vi "GetNI_SaveToFile.vi"(0 "Digitizer Settings":T5={"Digitizer delay (us) "=0.0, "rf points per line"=2048, "lines per plane"=128, "Samp Rate (Hz)"=100000000.0, "Additional dig delay (us)"=0.0, "Voltage Scale"=0.4, "Pre-Looks"=0, "Offset delay (us)"=0.0, "bits A/D"=8, "Avg Num"=1, "DigTimeOut"=5.0, "Rel Dig Delay"=0.0, "Dig Ch"=0, "LeCroyCluster"={"LeCroy Channels"=[TRUE, FALSE, FALSE, FALSE], "LC read pt offset"=0.0, "Sweep Avg"=FALSE}, "Main Digitizer"=enum."NI Digitizer", "Dig Config"=enum."Single channel", "Digitizer ID Cluster"={"Acqiris/Alazar/SP ID"=[], "NI Instr Handles"=[], "LeCroy VISA"="", "GaGe Handle"={"Handle"=0, "Sample size"=0, "Resolution"=0, "Offset"=0, "Channels"=0, "Boards"=0}, "ATS Ref"="ATS9350", "Acqiris Address"=["PCI::INSTR0"], "ADQRef"=refnum, "adq_cu_ptr"=refnum}, "Trigger Settings"={"Trig Source"=1, "Trig Coupling"=0, "Trig Slope"=0, "Level (mV)"=1500.0}, "Bulk Acq"=FALSE, "Bulk Start Indexes"=[], "Data Ref RF"=refnum, "NI ID/Channel"=[], "Total Dig CH"=1, "Xtra Ann Trig delay (us)"=10.0, "Fix Z Delay?"=FALSE, "One Way Transmission?"=FALSE, "Data Ref Log"=refnum} {"Trigger Settings"."Trig Slope" items=["Positive", "Negative"]; "Trigger Settings"."Level (mV)" format="%.2f"; "Trigger Settings"."Trig Coupling" items=["DC 1 MOhm", "AC 1 MOhm", "DC 50 Ohm", "AC 50 Ohm"]; "Trigger Settings"."Trig Source" items=["Chan 1", "External"]; "Rel Dig Delay" format="%.2f"; "DigTimeOut" format="%.2f"; "Avg Num" min=1; "Offset delay (us)" format="%.2f"; "Additional dig delay (us)" format="%.2f"; "Digitizer delay (us)" format="%.2f"}, 3 "NI Card":refnum<k15>, 6 "Motion Settings":T1={"No Motion?"=FALSE, "Motion System"=enum."NI 735x", "Motion Bd ID"=1, "Motion Profile"="SMAC1", "# Axis"=1, "Reverse Z axis?"=TRUE, "SMAC Axis"=0, "scan pair"=enum."y-(x) scan", "RT fps"=6.0, "Steps per mm"=[1000, 1000, 1000, 1000], "Motor Parameters"={"velocity ct/s"=[10000.0, 10000.0, 10000.0, 50000.0], "accel ct/s^2"=[50000.0, 50000.0, 50000.0, 200000.0]}, "One Way Scan"=FALSE, "Reverse One Way Scan"=FALSE, "Global Position (mm)"=[], "Plane"=0, "Distance between\nscan lines (um)"=0.0, "Distance between\nscan planes (um)"=0.0, "number of scan planes"=1, "Total steps in line"=0, "Xtra plane\ndistance  (um)"=100, "Xtra planes "=1, "Add Axis"=FALSE, "overshoot cts"=200, "BKPT Shift"=0, "Scan Start Time (ms)"=0, "ESP VISA"="GPIB::1::INSTR", "3rd Axis"=1, "GL Ref Out"=refnum, "Galil Address"=""} {"3rd Axis" items=["x", "y", "z", "w"]; "Xtra planes" min=1; "Xtra plane\ndistance  (um)" min=0; "Distance between\nscan planes (um)" format="%.2f"; "Distance between\nscan lines (um)" format="%.2f"; "SMAC Axis" items=["None"=0, "Axis 1"=1, "Axis 2"=2, "Axis 3"=3, "Axis 4"=4, "Axis 5"=5, "Axis 6"=6, "Axis 7"=7, "Axis 8"=8, "Vector Space 1"=17, "Vector Space 2"=18, "Vector Space 3"=19, "Vector Space 4"=20]; "Motion Bd ID" min=1 max=32 step=1}, 7 "errorin":errorcluster, 8 "File Array":string[](array[string]), 9 "Pulser Channel":i32, 10 "lines per plane":i32, 12 "Start Record":i32, 15 "Reverse?":bool) -> (17 "Raw VGain (scale)":dbl, 18 "Gain Array":T9(array[cluster]), 21 "VGain (dB)":dbl, 27 "error out":errorcluster)   [LabVIEW 2022 SP3]
uses:
  -DigitizerRoutines/DigitizerSettings.ctl
  -DigitizerRoutines/Digitizer.ctl
  -DigitizerRoutines/DigConfig.ctl
  -DigitizerRoutines/DigitizerID.ctl
  C:/Windows/System32/ADQAPI_dotNet_helper.dll
  Motion Controllers/NI_controller/-NI_MotionRoutines/MotionParameters.ctl
  Motion Controllers/NI_controller/-NI_MotionRoutines/MotionSys.ctl
  Motion Controllers/-MotionRoutines/ScanAxis.ctl
  Motion Controllers/-MotionRoutines/3rdAxis.ctl
  <instrlib>/niScope/Acquire/Fetch/niScope Multi Fetch Binary 8.vi
  -ScanSystem/DataHandling/ReverseDataI8.vi
panel:
  # "1-D and 2-D B scan settings"
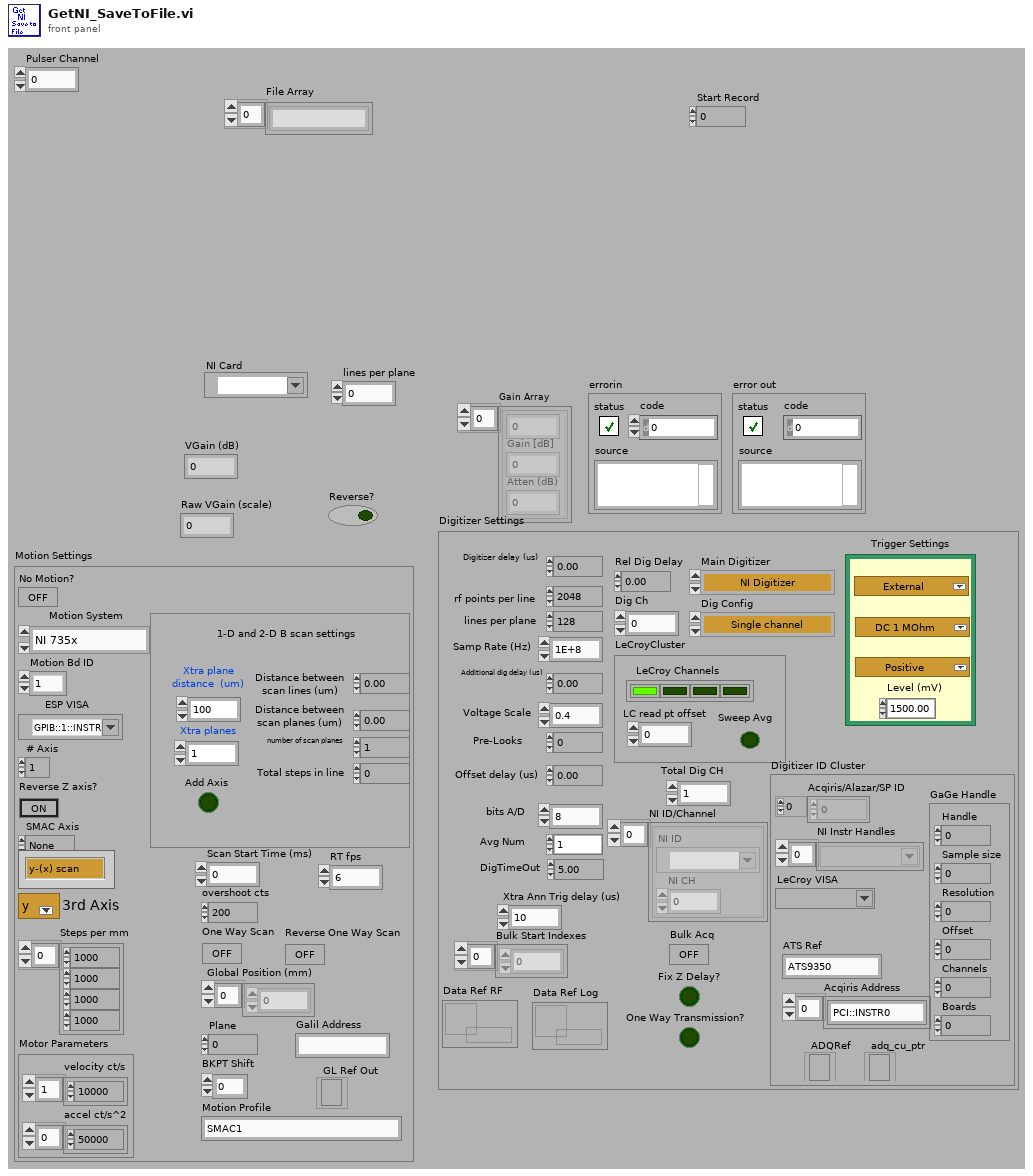
[diagram p1: front panel]
types:
  T1 = typedef "MotionParameters.ctl" = cluster{"No Motion?":bool, "Motion System":T2, "Motion Bd ID":u8, "Motion Profile":string, "# Axis":i8, "Reverse Z axis?":bool, "SMAC Axis":u16, "scan pair":T3, "RT fps":sgl, "Steps per mm":i32[], "Motor Parameters":cluster{"velocity ct/s":dbl[], "accel ct/s^2":dbl[]}, "One Way Scan":bool, "Reverse One Way Scan":bool, "Global Position (mm)":dbl[], "Plane":i32, "Distance between\nscan lines (um)":sgl, "Distance between\nscan planes (um)":sgl, "number of scan planes":i32, "Total steps in line":i32, "Xtra plane\ndistance  (um)":i32, "Xtra planes ":i32, "Add Axis":bool, "overshoot cts":i32, "BKPT Shift":i32, "Scan Start Time (ms)":u32, "ESP VISA":refnum<visa-resource-name>, "3rd Axis":T4, "GL Ref Out":refnum<k7>, "Galil Address":string}
  T2 = typedef "MotionSys.ctl" = enum16{"MM3000", "NI 735x", "Newport ESP", "No Motion Card", "Galil"}
  T3 = typedef "ScanAxis.ctl" = enum16{"y-(x) scan", "x-(y) scan", "z-(x) scan", "z-(y) scan", "y-(z) scan", "x-(z) scan", "w-(x) scan", "w-(y) scan", "w-(z) scan", "x-(w) scan", "y-(w) scan", "z-(w) scan"}
  T4 = typedef "3rdAxis.ctl" = u16
  T5 = typedef "DigitizerSettings.ctl" = cluster{"Digitizer delay (us) ":dbl, "rf points per line":i32, "lines per plane":i32, "Samp Rate (Hz)":dbl, "Additional dig delay (us)":dbl, "Voltage Scale":dbl, "Pre-Looks":i32, "Offset delay (us)":dbl, "bits A/D":i8, "Avg Num":i32, "DigTimeOut":sgl, "Rel Dig Delay":sgl, "Dig Ch":i32, "LeCroyCluster":cluster{"LeCroy Channels":bool[], "LC read pt offset":dbl, "Sweep Avg":bool}, "Main Digitizer":T6, "Dig Config":T7, "Digitizer ID Cluster":T8, "Trigger Settings":cluster{"Trig Source":u16, "Trig Coupling":u16, "Trig Slope":u16, "Level (mV)":dbl}, "Bulk Acq":bool, "Bulk Start Indexes":i32[], "Data Ref RF":refnum<data-value>, "NI ID/Channel":cluster{"NI ID":refnum<k15>, "NI CH":i32}[], "Total Dig CH":i32, "Xtra Ann Trig delay (us)":dbl, "Fix Z Delay?":bool, "One Way Transmission?":bool, "Data Ref Log":refnum<data-value>}
  T6 = typedef "Digitizer.ctl" = enum16{"Acqiris Digitizer", "NI Digitizer", "LeCroy", "GaGe", "AlazarTech", "No Digitizer", "Teledyne"}
  T7 = typedef "DigConfig.ctl" = enum16{"Single channel", "2 Chans w/ 2 Acqiris", "2 Chans w/ 1 Acqiris", "5-CH Pulser New", "5-CH pulser w/ ann array", "5-pass style ann array", "Empty"}
  T8 = typedef "DigitizerID.ctl" = cluster{"Acqiris/Alazar/SP ID":u32[], "NI Instr Handles":refnum<k15>[], "LeCroy VISA":refnum<visa-resource-name>, "GaGe Handle":cluster{"Handle":u32, "Sample size":u32, "Resolution":i32, "Offset":i32, "Channels":u32, "Boards":u32}, "ATS Ref":string, "Acqiris Address":string[], "ADQRef":refnum<k24>, "adq_cu_ptr":refnum<k24>}
  T9 = cluster{sgl, "Gain [dB]  ":sgl, "Atten (dB)":sgl}[]
  T10 = cluster{"actualSamples":i32, "absoluteInitialX":dbl, "relativeInitialX":dbl, "xIncrement":dbl, "offset":dbl, "gain":dbl, "reserved1":dbl, "reserved2":dbl}[]
  T11 = cluster{"actualSamples":i32, "absoluteInitialX":dbl, "relativeInitialX":dbl, "xIncrement":dbl, "offset":dbl, "gain":dbl, "reserved1":dbl, "reserved2":dbl}
  T12 = cluster{sgl, "Gain [dB]  ":sgl, "Atten (dB)":sgl}
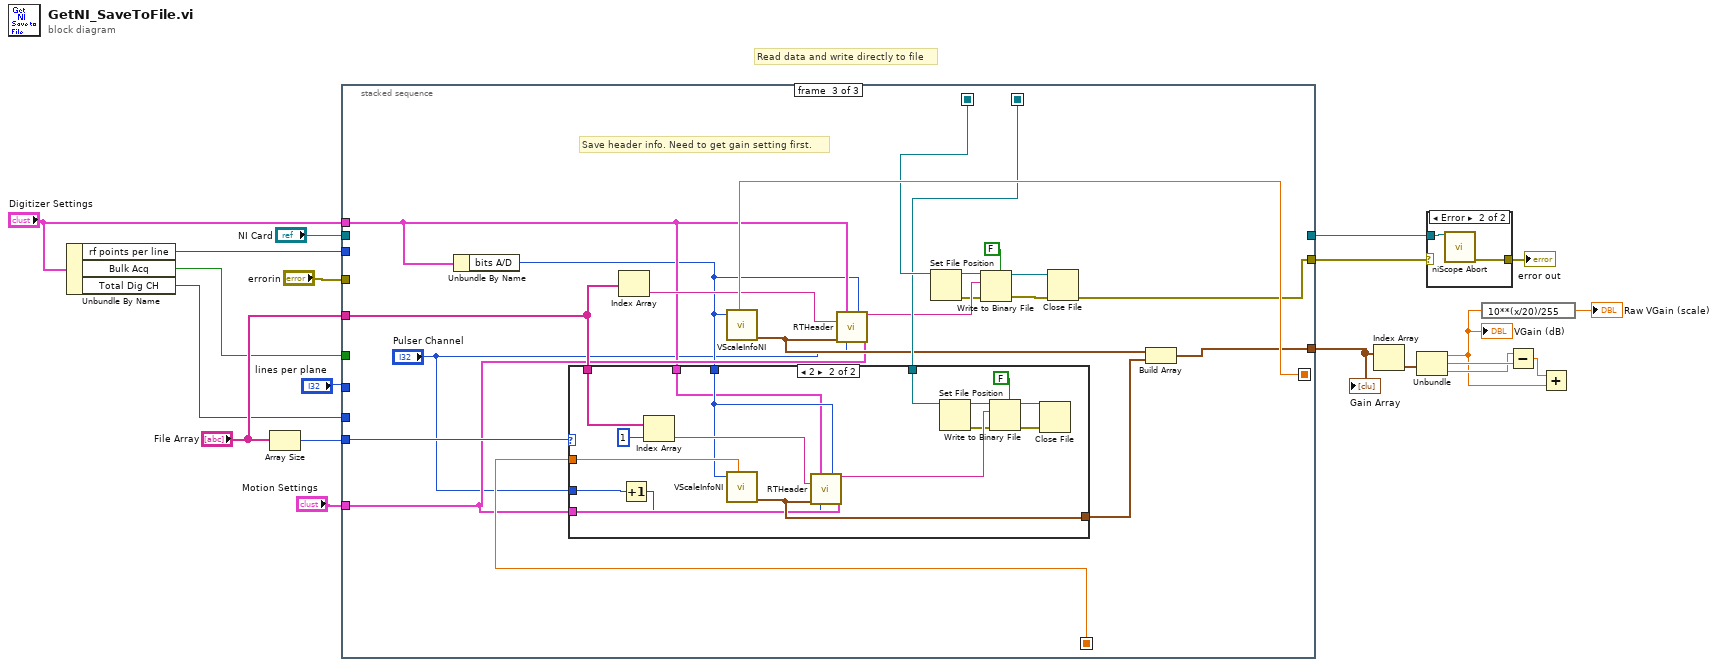
[diagram p0: block diagram]
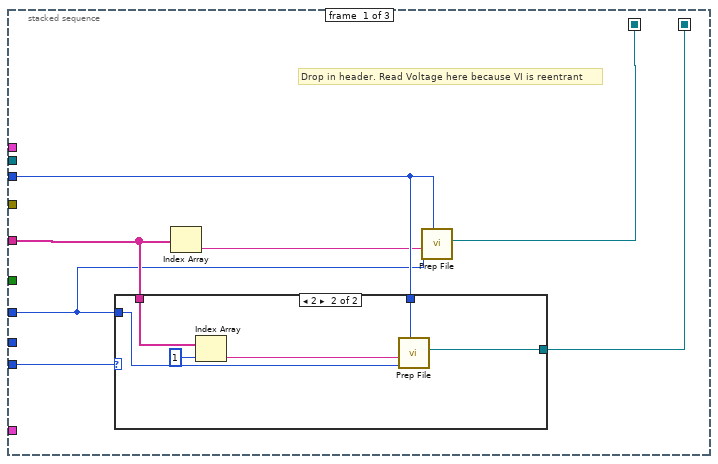
[diagram p2: hidden frame]
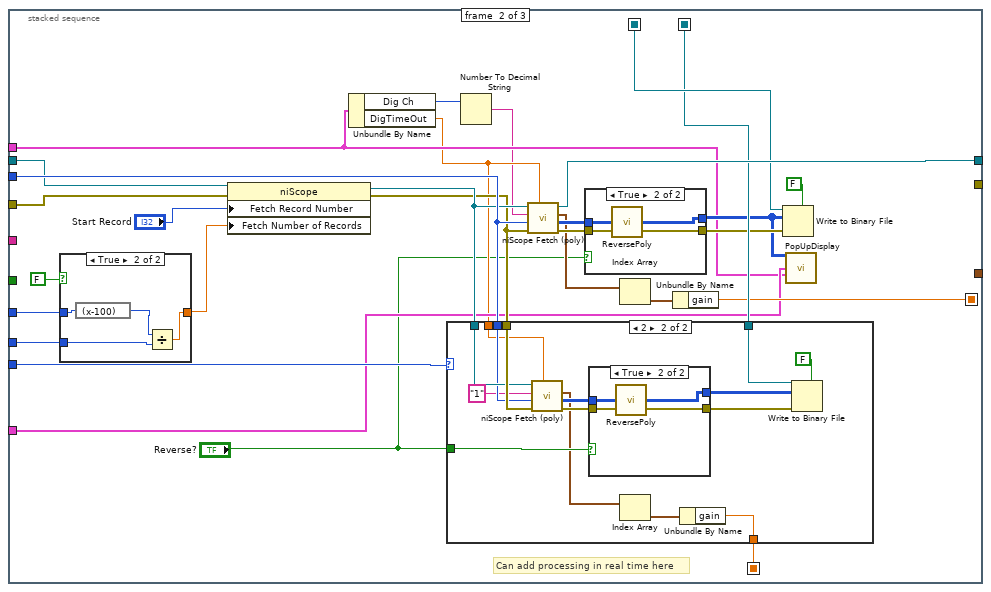
[diagram p4: hidden frame]
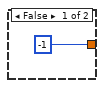
[diagram p8: hidden frame]
diagram:
  # "Read data and write directly to file"
  n1 = Unbundle By Name("Digitizer Settings") -> ("rf points per line"=w5:i32, "Bulk Acq"=w2:bool, "Total Dig CH"=w1:i32)
  n2 = Array Size(array="File Array") -> (size(s)=w13:i32)
  n3 = stacked-sequence {
    seq-local: [w27 _ _] -> [_ w60 w111]
    seq-local: [w22 _ _] -> [_ w53 w110]
    seq-local: [_ w51 _] -> [_ _ w112]
    seq-local: [_ w50 _] -> [_ _ w113]
    tunnel: [_ w62 _] -> w8
    tunnel: [_ _ w105] -> w7
    tunnel: "NI Card" -> [_ w57 _]
    tunnel: "lines per plane" -> [w24 w52 _]
    tunnel: w5 -> [w25 w61 _]
    tunnel: "File Array" -> [w26 _ w104]
    tunnel: "errorin" -> [_ w56 _]
    tunnel: w13 -> [w23 w54 w109]
    tunnel: [_ _ w106] -> w6
    tunnel: w2 -> [_ _ _]
    tunnel: "Digitizer Settings" -> [_ w39 w95]
    tunnel: "Motion Settings" -> [_ w40 w96]
    tunnel: w1 -> [_ w42 _]
    frame #0 {
      # "Drop in header. Read Voltage here because VI is reentrant"
      n4 = case shown="2" w23 {
        tunnel: w26 -> [_ w32]
        tunnel: [_ w31] -> w22
        tunnel: w24 -> [_ w29]
        tunnel: w25 -> [_ w28]
        frame 0, Default {
        }
        frame 2 {
          n5 = Index Array(array=w32, index=1) -> (element=w30:string)
          n6 = call "Prep File.vi"("Num Samps"=w28, "Num Segs"=w29, "File Name"=w30) -> ("refnum out"=w31:refnum<file>)  [unwired: 4 in, 1 out]
        }
      }
      n7 = Index Array(array=w26) -> (element=w21:string)  [unwired: 1 in]
      n8 = call "Prep File.vi"("Num Samps"=w25, "Num Segs"=w24, "File Name"=w21) -> ("refnum out"=w27:refnum<file>)  [unwired: 4 in, 1 out]
    }
    frame #1 {
      # "Can add processing in real time here"
      n9 = case shown="True" FALSE {
        tunnel: [-1 ("Fetch:Fetch Number of Records") w89] -> w55
        tunnel: w52 -> [_ w92]
        tunnel: w42 -> [_ w90]
        frame False {
        }
        frame True {
          n10 = expression code="(x-100)"(w92) -> (w91:i32)
          n11 = Divide(x=w91, y=w90) -> (x/y=w89:dbl)
        }
      }
      n12 = property class="niScope"(reference=w57, error in=w56, "Fetch Record Number"="Start Record", "Fetch Number of Records"=w55) -> (reference out=w59:refnum<k15>, error out=w58:errorcluster)
      n13 = Unbundle By Name(w39) -> ("Dig Ch"=w37:i32, "DigTimeOut"=w38:sgl)
      n14 = case shown="2" w54 {
        tunnel: w58 -> [_ w77]
        tunnel: w59 -> [_ w76]
        tunnel: w61 -> [_ w75]
        tunnel: "Reverse?" -> [_ w74]
        tunnel: w53 -> [_ w73]
        tunnel: w38 -> [_ w72]
        tunnel: [_ w63] -> w51
        frame 0, Default {
        }
        frame 2 {
          n15 = call-poly <instrlib>:"niScope Fetch (poly).vi"("timeout"=w72, "error in"=w77, "numSamples"=w75, "channels"="1", "instrument handle"=w76) -> ("error out"=w70:errorcluster, "wfm"=w71:i8[][], "wfm info"=w65:T10)  [unwired: 4 out]
          n16 = case shown="True" w74 {
            tunnel: [w79 w82] -> w66
            tunnel: w71 -> [w79 w81]
            tunnel: [w78 w80] -> w67
            tunnel: w70 -> [w78 w80]
            frame False {
            }
            frame True {
              n17 = call-poly "ReversePoly.vi"("Array in"=w81) -> ("Array out"=w82:i8[][])
            }
          }
          n18 = Index Array(array=w65) -> (element=w64:T11)  [unwired: 1 in]
          n19 = Unbundle By Name(w64) -> ("gain"=w63:dbl)
          n20 = Write to Binary File(file (use dialog)=w73, data=w66, error in=w67, 5:FALSE ("prepend array or string size? (T)")) -> ()  [unwired: 2 in, 3 out]
        }
      }
      n21 = Number To Decimal String(number=w37) -> (decimal integer string=w36:string)  [unwired: 1 out]
      n22 = call-poly <instrlib>:"niScope Fetch (poly).vi"("timeout"=w38, "error in"=w58, "numSamples"=w61, "channels"=w36, "instrument handle"=w59) -> ("error out"=w46:errorcluster, "wfm"=w49:i8[][], "wfm info"=w45:T10, "instrument handle out"=w62:refnum<k15>)  [unwired: 3 out]
      n23 = case shown="True" "Reverse?" {
        tunnel: [w84 w87] -> w41
        tunnel: w49 -> [w84 w86]
        tunnel: [w83 w85] -> w47
        tunnel: w46 -> [w83 w85]
        frame False {
        }
        frame True {
          n24 = call-poly "ReversePoly.vi"("Array in"=w86) -> ("Array out"=w87:i8[][])
        }
      }
      n25 = Index Array(array=w45) -> (element=w44:T11)  [unwired: 1 in]
      n26 = Unbundle By Name(w44) -> ("gain"=w50:dbl)
      n27 = Write to Binary File(file (use dialog)=w60, data=w41, error in=w47, 5:FALSE ("prepend array or string size? (T)")) -> ()  [unwired: 2 in, 3 out]
      n28 = call "PopUpDisplay.vi"("Data"=w41, "Motion Settings In"=w40, "Digitizer Settings"=w39) -> ()  [unwired: 13 in]
    }
    frame #2 {
      # "Save header info. Need to get gain setting first."
      n29 = Unbundle By Name(w95) -> ("bits A/D"=w94:i8)
      n30 = case shown="2" w109 {
        tunnel: w112 -> [_ w127]
        tunnel: w110 -> [_ w123]
        tunnel: [_ w122] -> w107
        tunnel: w104 -> [_ w120]
        tunnel: w94 -> [_ w118]
        tunnel: w95 -> [_ w117]
        tunnel: w96 -> [_ w116]
        tunnel: "Pulser Channel" -> [_ w115]
        frame 0, Default {
        }
        frame 2 {
          n31 = Increment(x=w115) -> (x+1=w114:i32)
          n32 = Index Array(array=w120, index=1) -> (element=w119:string)
          n33 = call "VScaleInfoNI.vi"("A/D bits"=w118, "gain"=w127) -> ("Voltage Scale"=w122:T12)  [unwired: 5 in, 3 out]
          n34 = call "RTHeader.vi"("Digitizer Settings"=w117, "Dig Word Size"=w118, "File Name In"=w119, "Votage scaling"=w122, "Pulser Channel"=w114, "Motion Settings"=w116) -> ("Header String Out"=w126:string)  [unwired: 8 in, 1 out]
          n35 = Set File Position(refnum=w123) -> (refnum out=w125:refnum<file>, error out=w124:errorcluster)  [unwired: 3 in]
          n36 = Write to Binary File(file (use dialog)=w125, data=w126, error in=w124, 5:FALSE ("prepend array or string size? (T)")) -> (refnum out=w128:refnum<file>, error out=w129:errorcluster)  [unwired: 2 in, 1 out]
          n37 = Close File(refnum=w128, error in=w129) -> ()  [unwired: 2 out]
        }
      }
      n38 = Index Array(array=w104) -> (element=w97:string)  [unwired: 1 in]
      n39 = call "VScaleInfoNI.vi"("A/D bits"=w94, "gain"=w113) -> ("Voltage Scale"=w108:T12)  [unwired: 5 in, 3 out]
      n40 = call "RTHeader.vi"("Digitizer Settings"=w95, "Dig Word Size"=w94, "File Name In"=w97, "Votage scaling"=w108, "Pulser Channel"="Pulser Channel", "Motion Settings"=w96) -> ("Header String Out"=w100:string)  [unwired: 8 in, 1 out]
      n41 = Set File Position(refnum=w111) -> (refnum out=w99:refnum<file>, error out=w98:errorcluster)  [unwired: 3 in]
      n42 = Write to Binary File(file (use dialog)=w99, data=w100, error in=w98, 5:FALSE ("prepend array or string size? (T)")) -> (refnum out=w102:refnum<file>, error out=w101:errorcluster)  [unwired: 2 in, 1 out]
      n43 = Close File(refnum=w102, error in=w101) -> (error out=w105:errorcluster)  [unwired: 1 out]
      n44 = Build Array(w108, w107) -> (w106:T9)
    }
  }
  "Gain Array" <- w6
  n45 = Index Array(array=w6) -> (element=w15:T12)  [unwired: 1 in]
  n46 = Unbundle(w15) -> (w16:sgl, "Gain [dB]"=w18:sgl, "Atten (dB)"=w17:sgl)
  "VGain (dB)" <- w16
  n47 = case shown="Error" w7 {
    selector: w7 -> [w131 _]
    tunnel: w8 -> [_ w133]
    tunnel: [w131 w132] -> w14
    frame No Error {
    }
    frame Error {
      n48 = call <instrlib>:"niScope Abort.vi"("instrument handle"=w133) -> ("error out"=w132:errorcluster)  [unwired: 1 in, 13 out]
    }
  }
  "error out" <- w14
  n49 = expression code="10**(x/20)/255"(w16) -> (→"Raw VGain (scale)":sgl)
  n50 = Subtract(x=w17, y=w18) -> (x-y=w19:sgl)
  n51 = Add(x=w19, y=w16) -> ()  [unwired: 1 out]
